vi "trim history.vi"(5 "Values":dbl[][](array[numeric]), 9 "Timestamps":dbl[][](array[numeric])) -> (8 "Array 3":cluster{dbl[], dbl[]}[](array[cluster]))   [LabVIEW 2018]
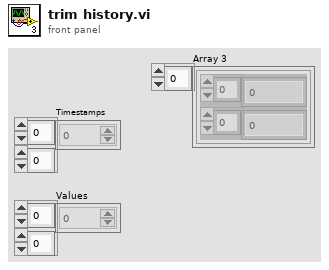
[diagram p1: front panel]
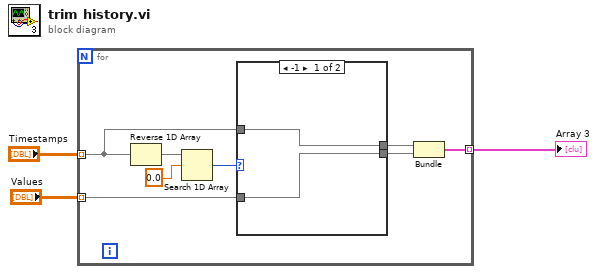
[diagram p0: block diagram]
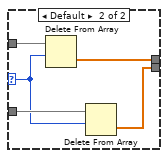
[diagram p2: hidden frame]
diagram:
  n1 = for {
    tunnel: "Values" -> [w8] mode=indexing
    tunnel: [w11] -> w1 mode=indexing
    tunnel: "Timestamps" -> [w4] mode=indexing
    n2 = Reverse 1D Array(array=w4) -> (reversed array=w10:dbl[])
    n3 = Search 1D Array(1D array=w10, element=0.0) -> (index of element=w5:i32)  [unwired: 1 in]
    n4 = case shown="-1" w5 {
      selector: w5 -> [_ w16]
      tunnel: w8 -> [w13 w18]
      tunnel: [w13 w14] -> w7
      tunnel: [w12 w15] -> w6
      tunnel: w4 -> [w12 w17]
      frame -1 {
      }
      frame Default {
        n5 = Delete From Array(array=w17, length=w16) -> (deleted portion=w15:dbl[])  [unwired: 1 in, 1 out]
        n6 = Delete From Array(array=w18, length=w16) -> (deleted portion=w14:dbl[])  [unwired: 1 in, 1 out]
      }
    }
    n7 = Bundle("Timestamps"=w6, "Values"=w7) -> (w11:cluster{"Timestamps":dbl[], "Values":dbl[]})  [unwired: 1 in]
  }
  "Array 3" <- w1
